vi "gaussian wave function.vi"(0 "t us":dbl, 1 "f MHz":dbl, 2 "phase0 pi":dbl, 12 "peak position us":dbl, 13 "sd us":dbl) -> (4 "Result":dbl)   [LabVIEW 2020]
uses:
  <vilib>/express/express arith-compare/Formula/XNode/ExpressFormulaBlockNode.xnode
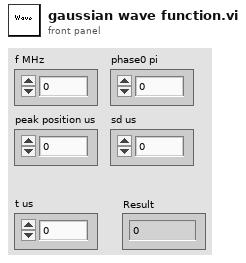
[diagram p1: front panel]
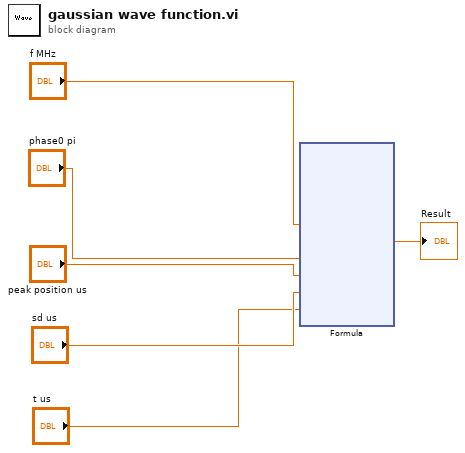
[diagram p0: block diagram]
diagram:
  n1 = xnode "Formula"("f"="f MHz", "p0"="phase0 pi", "u"="peak position us", "sd"="sd us", "t"="t us") -> ("Result"=→"Result":dbl)  [unwired: 1 in, 1 out]
